vi "AdcConversion.vi"(8 "error in (no error)":errorcluster, 11 "Single Channel ADC in":refnum<class "Single Channel ADC.lvclass">) -> (0 "error out":errorcluster, 2 "ADC U8 Array":u8[](array[numeric]), 3 "Single Channel ADC out":refnum<class "Single Channel ADC.lvclass">)   [LabVIEW 2023, in "Single Channel ADC.lvclass"]
uses:
  Single Channel ADC.lvclass
  <vilib>/numeric/Random Number (Range) U64.vi
  <vilib>/numeric/sub_Random U32.vi
  Single Channel ADC.lvclass/Single Channel ADC.ctl
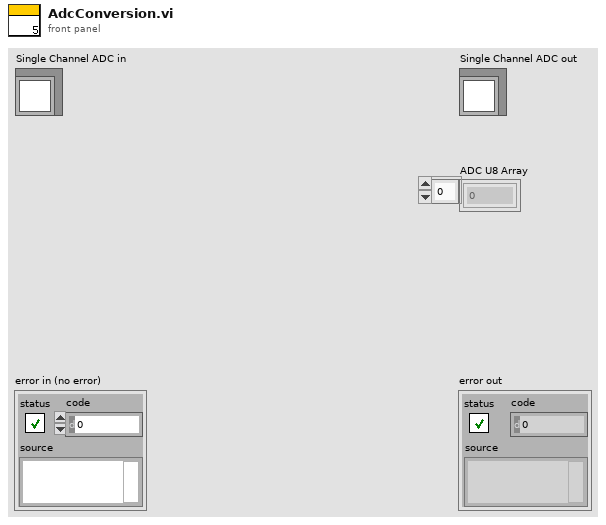
[diagram p1: front panel]
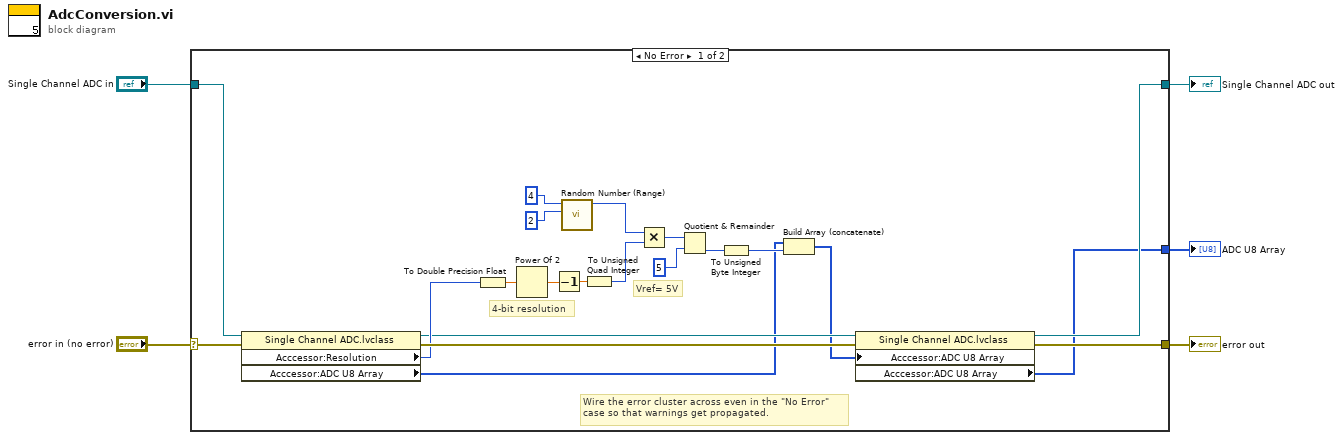
[diagram p0: block diagram]
diagram:
  n1 = case shown="No Error" "error in (no error)" {
    selector: "error in (no error)" -> [w26 w28]
    tunnel: [w12 w28] -> w4
    tunnel: [w9 w27] -> w2
    tunnel: "Single Channel ADC in" -> [w10 w27]
    tunnel: [w6 _] -> w1
    frame No Error {
      # "Vref= 5V"
      # "4-bit resolution"
      # "Wire the error cluster across even in the \"No Error\"\ncase so that warnings get propagated."
      n2 = property class="Single Channel ADC.lvclass"(reference=w10, error in=w26) -> (reference out=w11:refnum<class "Single Channel ADC.lvclass">, error out=w14:errorcluster, "Acccessor:Resolution"=w13:i32, "Acccessor:ADC U8 Array"=w8:u8[])
      n3 = To Double Precision Float(number=w13) -> (double precision float=w18:dbl)
      n4 = Power Of 2(x=w18) -> (2^x=w20:dbl)
      n5 = Decrement(x=w20) -> (x-1=w25:dbl)
      n6 = call-poly <vilib>:"Random Number (Range).vi"("lower bound (0)"=u64 2, "upper bound (100)"=u64 4) -> ("number"=w15:u64)  [unwired: 9 in]
      n7 = To Unsigned Quad Integer(1:w25) -> (0:w19:u64)
      n8 = Multiply(x=w15, y=w19) -> (x*y=w23:u64)
      n9 = Quotient & Remainder(x=w23, y=u64 5 ("upper bound (100)")) -> (floor(x/y)=w22:u64)  [unwired: 1 out]
      n10 = To Unsigned Byte Integer(number=w22) -> (unsigned 8bit integer=w21:u8)
      n11 = Build Array (concatenate)(w8, w21) -> (w7:u8[])
      n12 = property class="Single Channel ADC.lvclass"(reference=w11, error in=w14, "Acccessor:ADC U8 Array"=w7) -> (reference out=w9:refnum<class "Single Channel ADC.lvclass">, error out=w12:errorcluster, "Acccessor:ADC U8 Array"=w6:u8[])
    }
    frame Error {
    }
  }
  "error out" <- w4
  "Single Channel ADC out" <- w2
  "ADC U8 Array" <- w1
